vi "Get IRF support & Guess Values.vi"(6 "Fraction of Original Support (0.7)":dbl=0.7, 8 "error in (no error)":errorcluster, 10 "IRF Array in":dbl[](array[numeric]), 11 "t Array in":dbl[](array[numeric])) -> (0 "error out":errorcluster, 2 "IRF Array out":dbl[](array[numeric]), 3 "t Array out":dbl[](array[numeric]))   [LabVIEW 2021, in "Fits.lvlib"]
uses:
  Fits.lvlib
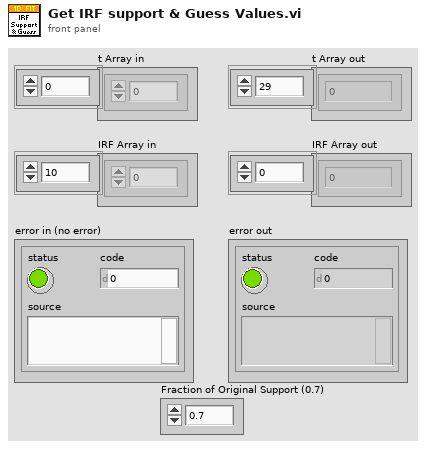
[diagram p1: front panel]
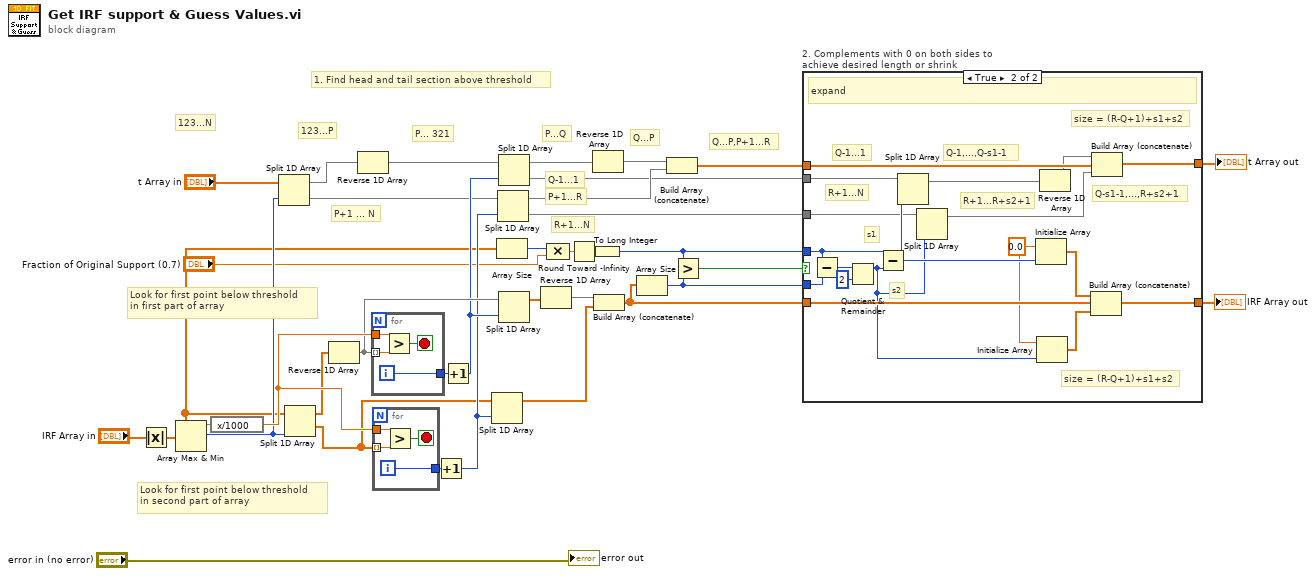
[diagram p0: block diagram]
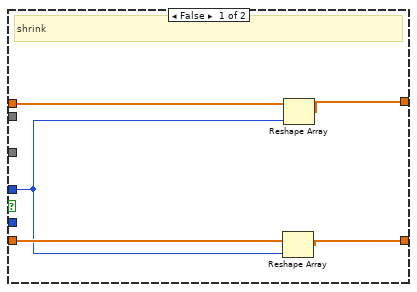
[diagram p2: hidden frame]
diagram:
  # "R+1...N"
  # "Q...P,P+1...R"
  # "Q...P"
  # "P+1...R"
  # "Q-1...1"
  # "P...Q"
  # "P... 321"
  # "P+1 ... N"
  # "123...P"
  # "123...N"
  # "1. Find head and tail section above threshold"
  # "Look for first point below threshold\nin second part of array"
  # "Look for first point below threshold\nin first part of array"
  n1 = Absolute Value(x="IRF Array in") -> (abs(x)=w12:dbl[])
  n2 = Array Max & Min(array=w12) -> (max value=w35:dbl, max index (indices)=w32:i32)  [unwired: 2 out]
  n3 = expression code="x/1000"(w35) -> (w34:dbl)
  n4 = Split 1D Array(array="t Array in", index=w32) -> (first subarray=w31:dbl[], second subarray=w23:dbl[])
  n5 = Split 1D Array(array=w12, index=w32) -> (first subarray=w19:dbl[], second subarray=w17:dbl[])
  n6 = Reverse 1D Array(array=w19) -> (reversed array=w27:dbl[])
  n7 = Reverse 1D Array(array=w31) -> (reversed array=w30:dbl[])
  n8 = for {
    tunnel: w27 -> [w39] mode=indexing
    tunnel: w34 -> [w40]
    tunnel: [w37] -> w26
    i -> [w37]
    stop <- w38 stop-if-true
    n9 = Greater?(x=w40, y=w39) -> (0:w38:bool)
  }
  n10 = for {
    tunnel: w17 -> [w43] mode=indexing
    tunnel: w34 -> [w44]
    tunnel: [w41] -> w25
    i -> [w41]
    stop <- w42 stop-if-true
    n11 = Greater?(x=w44, y=w43) -> (0:w42:bool)
  }
  n12 = Increment(x=w25) -> (x+1=w22:i32)
  n13 = Increment(x=w26) -> (x+1=w24:i32)
  n14 = Split 1D Array(array=w17, index=w22) -> (first subarray=w16:dbl[])  [unwired: 1 out]
  n15 = Array Size(array=w12) -> (size(s)=w13:i32)
  n16 = Split 1D Array(array=w23, index=w22) -> (first subarray=w21:dbl[], second subarray=w1:dbl[])
  n17 = Split 1D Array(array=w30, index=w24) -> (first subarray=w29:dbl[], second subarray=w2:dbl[])
  n18 = Split 1D Array(array=w27, index=w24) -> (first subarray=w18:dbl[])  [unwired: 1 out]
  n19 = Reverse 1D Array(array=w18) -> (reversed array=w15:dbl[])
  n20 = Compound Arithmetic op=MULTIPLY(w13, "Fraction of Original Support (0.7)") -> (w11:dbl)
  n21 = Round Toward -Infinity(1:w11) -> (0:w10:dbl)
  n22 = To Long Integer(number=w10) -> (32bit integer=w6:i32)
  n23 = Reverse 1D Array(array=w29) -> (reversed array=w28:dbl[])
  n24 = Build Array (concatenate)(w15, w16) -> (w8:dbl[])
  n25 = Array Size(array=w8) -> (size(s)=w3:i32)
  n26 = Build Array (concatenate)(w28, w21) -> (w7:dbl[])
  n27 = Greater?(x=w6, y=w3) -> (0:w9:bool)
  n28 = case "2. Complements with 0 on both sides to achieve desired length or shrink" shown="True" w9 {
    tunnel: w8 -> [w48 w63]
    tunnel: w7 -> [w49 w59]
    tunnel: w6 -> [w47 w64]
    tunnel: [w46 w58] -> w5
    tunnel: [w45 w60] -> w4
    tunnel: w3 -> [_ w67]
    tunnel: w2 -> [_ w57]
    tunnel: w1 -> [_ w52]
    frame False {
      # "shrink"
      n29 = Reshape Array(w48, w47) -> (w45:dbl[])
      n30 = Reshape Array(w49, w47) -> (w46:dbl[])
    }
    frame True {
      w53 = 0.0 ("element")
      # "size = (R-Q+1)+s1+s2"
      # "size = (R-Q+1)+s1+s2"
      # "Q-s1-1,...,R+s2+1"
      # "R+1...R+s2+1"
      # "R+1...N"
      # "s2"
      # "s1"
      # "Q-1,...,Q-s1-1"
      # "Q-1...1"
      # "expand"
      n31 = Subtract(x=w64, y=w67) -> (x-y=w66:i32)
      n32 = Quotient & Remainder(x=w66, y=2) -> (x-y*floor(x/y)=w51:i32)  [unwired: 1 out]
      n33 = Subtract(x=w64, y=w51) -> (x-y=w56:i32)
      n34 = Split 1D Array(array=w57, index=w56) -> (first subarray=w55:dbl[])  [unwired: 1 out]
      n35 = Split 1D Array(array=w52, index=w51) -> (first subarray=w50:dbl[])  [unwired: 1 out]
      n36 = Initialize Array(w53, w56) -> (w61:dbl[])
      n37 = Initialize Array(w53, w51) -> (w62:dbl[])
      n38 = Reverse 1D Array(array=w55) -> (reversed array=w54:dbl[])
      n39 = Build Array (concatenate)(w61, w63, w62) -> (w60:dbl[])
      n40 = Build Array (concatenate)(w54, w59, w50) -> (w58:dbl[])
    }
  }
  "IRF Array out" <- w4
  "t Array out" <- w5
  "error out" <- "error in (no error)"
